vi "ClassPanel.vi"(8 "error in (no error)":errorcluster caption="entrée d'erreur (pas d'erreur)", 11 "DefaultDev.lvclass":refnum<class "Calculations.lvclass">) -> (0 "error out":errorcluster caption="sortie d'erreur", 3 "DefaultDev.lvclass Out":refnum<class "Calculations.lvclass">)   [LabVIEW 2012, in "Calculations.lvclass"]
uses:
  Calculations.lvclass
  DevicesClass/BaseDevice/Accessor/GetClassEvent.vi
panel:
  in  "Stop":bool
  out "2":dbl format="%<%H:%M:%S%1u>t"
  in  "MiseAJour":bool
  in  "1":dbl=60.0 min=0.1 step=0.1 format="%#.1f"
  out "Init Program":bool
  # "this MUST labeled with class name"
  # "this MUST be present and labeled \"Stop\""
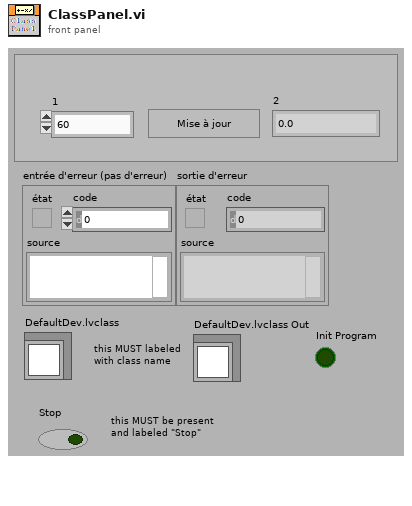
[diagram p1: front panel]
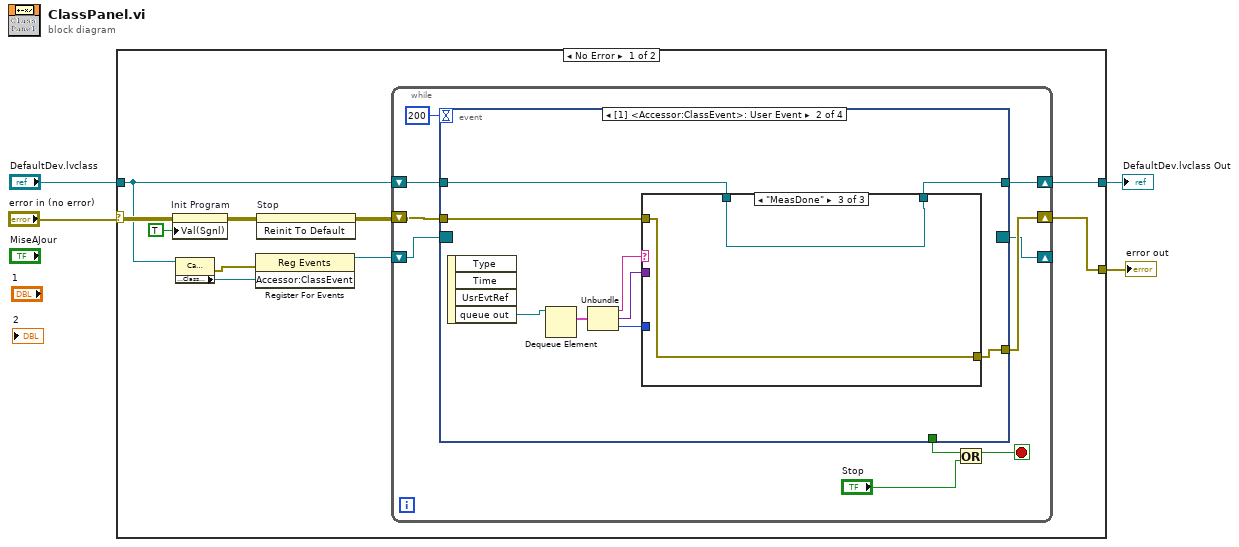
[diagram p0: block diagram]
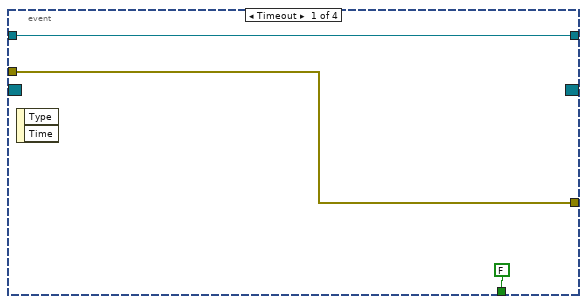
[diagram p2: hidden frame]
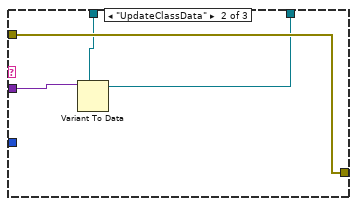
[diagram p4: hidden frame]
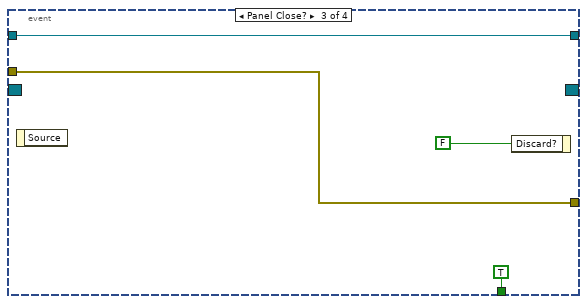
[diagram p5: hidden frame]
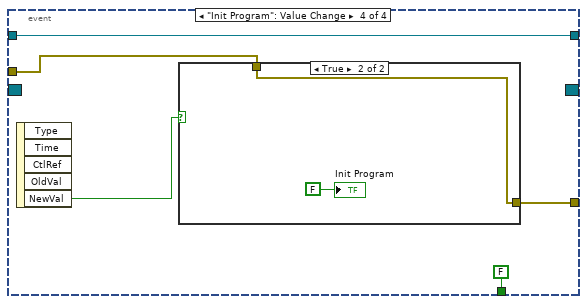
[diagram p6: hidden frame]
diagram:
  n1 = case shown="No Error" "error in (no error)" {
    selector: "error in (no error)" -> [w11 w58]
    tunnel: [w14 w58] -> w3
    tunnel: "DefaultDev.lvclass" -> [w6 w57]
    tunnel: [w12 w57] -> w1
    frame No Error {
      n2 = property on="Init Program" class="Bool (strict)"(error in=w11, "Val(Sgnl)"=TRUE ("Valeur (Signalisation)")) -> (error out=w10:errorcluster)  [unwired: 1 in, 1 out]
      n3 = property class="Calculations.lvclass"(reference=w6) -> (error out=w8:errorcluster, "Accessor:ClassEvent"=w7:refnum<user-event>)  [unwired: 1 in, 1 out]
      n4 = register-events(error in=w8, w7) -> (reference out=w5:refnum<event-registration>)  [unwired: 1 in, 1 out]
      n5 = invoke on="Stop" class="Bool (strict)" method="Reinit To Default"(error in=w10) -> (error out=w9:errorcluster)  [unwired: 2 in, 2 out]
      n6 = while {
        shift-right: [w22] -> w14
        shift-left: w9 -> [w23]
        shift-right: [w19] -> w12
        shift-left: w6 -> [w21]
        shift-right: [w15] -> _
        shift-left: w5 -> [w16]
        stop <- w18 stop-if-true
        n7 = event shown="[1] <Accessor:ClassEvent>: User Event" {
          selector: w16 -> [_ _ _ _]
          dyn-events: [_ _ _ _] -> w15
          timeout: 200 -> [_ _ _ _]
          tunnel: w23 -> [w25 w35 w46 w52]
          tunnel: [w25 w29 w46 w51] -> w22
          tunnel: w21 -> [w26 w36 w45 w50]
          tunnel: [FALSE _ TRUE FALSE] -> w20
          tunnel: [w26 w28 w45 w50] -> w19
          event Timeout {
            n8 = event-data() -> ()  [unwired: 1 in, 2 out]
          }
          event User Event {
            n9 = event-data() -> ("queue out"=w33:refnum<queue>)  [unwired: 1 in, 3 out]
            n10 = Dequeue Element(queue=w33) -> (element=w34:cluster{"Message":string, "Data":variant, i32})  [unwired: 2 in, 3 out]
            n11 = Unbundle(w34) -> ("Message"=w32:string, "Data"=w31:variant, w30:i32)
            n12 = case shown="\"MeasDone\"" w32 {
              tunnel: w35 -> [w38 w42 w43]
              tunnel: w31 -> [_ w41 _]
              tunnel: w36 -> [w37 w40 w44]
              tunnel: [w37 w39 w44] -> w28
              tunnel: [w38 w42 w43] -> w29
              tunnel: w30 -> [_ _ _]
              frame Default {
              }
              frame "UpdateClassData" {
                n13 = Variant To Data(type=w40, Variant=w41) -> (data=w39:refnum<class "Calculations.lvclass">)  [unwired: 1 in, 1 out]
              }
              frame "MeasDone" {
              }
            }
          }
          event Panel Close? {
            n14 = event-data() -> ()  [unwired: 1 in, 1 out]
            n15 = event-data("Discard?"=FALSE ("Rejeter ?")) -> ()  [unwired: 1 in, 1 out]
          }
          event "Init Program": Value Change {
            n16 = event-data() -> ("NewVal"=w53:bool)  [unwired: 1 in, 4 out]
            n17 = case shown="True" w53 {
              tunnel: w52 -> [w54 w55]
              tunnel: [w54 w55] -> w51
              frame False {
              }
              frame True {
                "Init Program" <- FALSE
              }
            }
          }
        }
        n18 = Or(x=w20, y="Stop") -> (x .or. y?=w18:bool)
      }
    }
    frame Error {
    }
  }
  "error out" <- w3
  "DefaultDev.lvclass Out" <- w1
